vi "Get queryserver_TestDataTypesParameters.vi"(8 "error in (no error)":errorcluster, 11 "gRPCid":T4) -> (0 "error out":errorcluster, 2 "Message Data":T1, 3 "gRPCid out":T4)   [LabVIEW 2019, in "TestDataMarshal.lvlib" / "TestDataMarshal.lvclass"]
uses:
  TestDataMarshal.lvclass
  gRPC lvSupport/Server API/typeDefs/grpcId.ctl
  queryserver_TestDataTypesParameters_Data.ctl
  queryserver_DataTypeTest/queryserver_DataTypeTest_Data.ctl
  google_protobuf_Any/google_protobuf_Any_Data.ctl
  a51dd2a7-b5c1-4c09-9df4-8cd9d3bd0c19.vi
  gRPC lvSupport/Server API/Server/Get Server DLL Path.vi
  gRPC lvSupport/gprc-lvsupport.lvlib
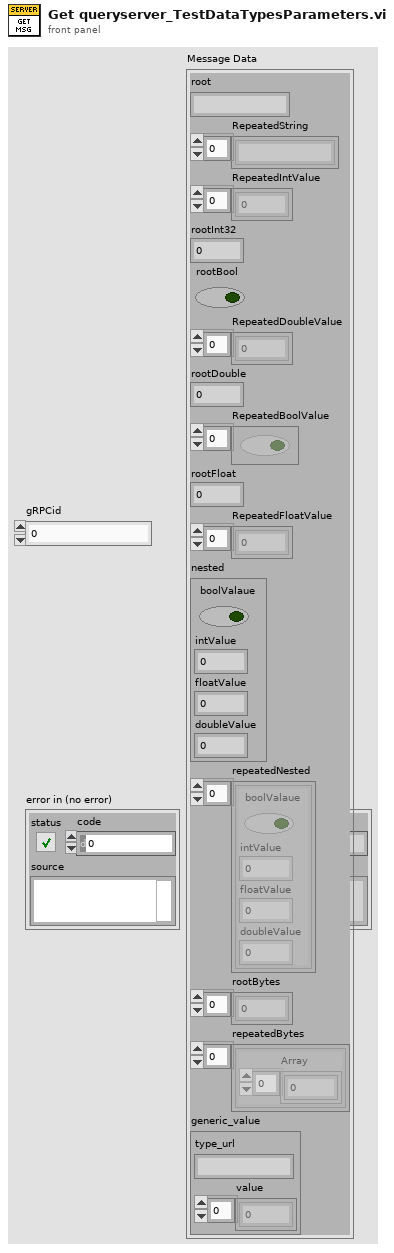
[diagram p1: front panel]
types:
  T1 = typedef "TestDataMarshal.lvlib/TestDataMarshal.lvclass/queryserver_TestDataTypesParameters_Data.ctl" = cluster{"root":string, "RepeatedString":string[], "RepeatedIntValue":i32[], "rootInt32":i32, "rootBool":bool, "RepeatedDoubleValue":dbl[], "rootDouble":dbl, "RepeatedBoolValue":bool[], "rootFloat":sgl, "RepeatedFloatValue":sgl[], "nested":T2, "repeatedNested":T2[], "rootBytes":u8[], "repeatedBytes":cluster{"Array":u8[]}[], "generic_value":T3}
  T2 = typedef "TestDataMarshal.lvlib/TestDataMarshal.lvclass/queryserver_DataTypeTest_Data.ctl" = cluster{"boolValaue":bool, "intValue":i32, "floatValue":sgl, "doubleValue":dbl}
  T3 = typedef "TestDataMarshal.lvlib/TestDataMarshal.lvclass/google_protobuf_Any_Data.ctl" = cluster{"type_url":string, "value":u8[]}
  T4 = typedef "TestDataMarshal.lvlib/gprc-lvsupport.lvlib/grpcId.ctl" = u64
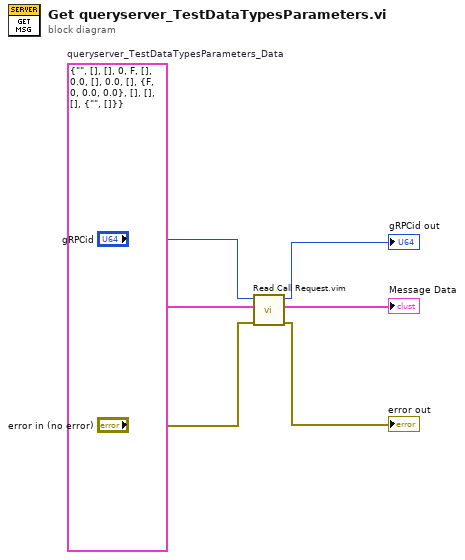
[diagram p0: block diagram]
diagram:
  w2 = T1 {"root"="", "RepeatedString"=[], "RepeatedIntValue"=[], "rootInt32"=0, "rootBool"=FALSE, "RepeatedDoubleValue"=[], "rootDouble"=0.0, "RepeatedBoolValue"=[], "rootFloat"=0.0, "RepeatedFloatValue"=[], "nested"={"boolValaue"=FALSE, "intValue"=0, "floatValue"=0.0, "doubleValue"=0.0}, "repeatedNested"=[], "rootBytes"=[], "repeatedBytes"=[], "generic_value"={"type_url"="", "value"=[]}}  # queryserver_TestDataTypesParameters_Data
  n1 = call "Read Call Request.vim"("error in (no error)"="error in (no error)", "Data Type"=w2, "gRPCid in"="gRPCid") -> ("error out"=→"error out":errorcluster, "Request Data"=→"Message Data":T1, "gRPCid out"=→"gRPCid out":T4)  [unwired: 6 in]
